vi "FN.vi"(0 "Offset_h":dbl, 1 "Offset_out":dbl, 2 "Inputs":dbl[](array[numeric]), 3 "Weights_h":dbl[][](array[numeric]), 4 "Weights_out":dbl[][](array[numeric])) -> (5 "Outputs_hx":dbl[](array[numeric]), 6 "Outputs_out":dbl[](array[numeric]))   [LabVIEW 2016]
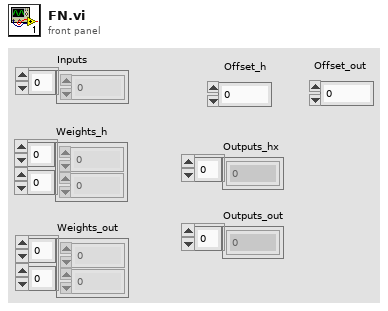
[diagram p1: front panel]
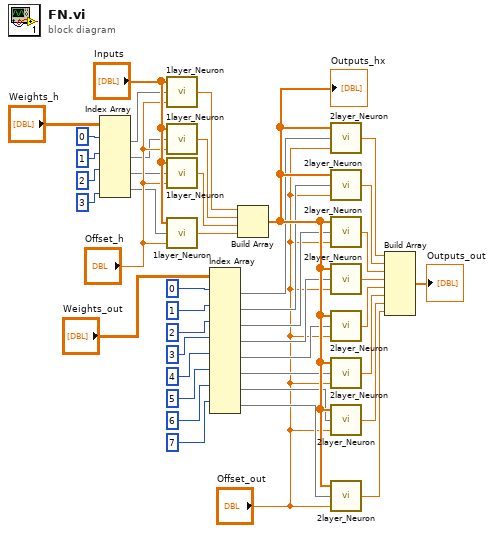
[diagram p0: block diagram]
diagram:
  n1 = Index Array(array="Weights_h", index (row) #1=0 ("index (row)"), index (row) #2=1 ("index (row)"), index (row) #3=2 ("index (row)"), index (col) #4=3 ("disabled index (col)")) -> (element #1=w31:dbl[], element #2=w30:dbl[], element #3=w29:dbl[], element #4=w28:dbl[])  [unwired: 4 in]
  n2 = call "1layer_Neuron.vi"("Offset"="Offset_h", "Weights"=w31, "Inputs"="Inputs") -> ("Output"=w41:dbl)
  n3 = call "1layer_Neuron.vi"("Offset"="Offset_h", "Weights"=w30, "Inputs"="Inputs") -> ("Output"=w40:dbl)
  n4 = call "1layer_Neuron.vi"("Offset"="Offset_h", "Weights"=w29, "Inputs"="Inputs") -> ("Output"=w39:dbl)
  n5 = call "1layer_Neuron.vi"("Offset"="Offset_h", "Weights"=w28, "Inputs"="Inputs") -> ("Output"=w38:dbl)
  n6 = Index Array(array="Weights_out", index (row) #1=0 ("index (row)"), index (row) #2=1 ("index (row)"), index (row) #3=2 ("index (row)"), index (row) #4=3 ("disabled index (col)"), index (row) #5=4 ("index (row)"), index (row) #6=5 ("index (row)"), index (row) #7=6 ("index (row)"), index (row) #8=7 ("disabled index (col)")) -> (element #1=w18:dbl[], element #2=w17:dbl[], element #3=w16:dbl[], element #4=w15:dbl[], element #5=w14:dbl[], element #6=w13:dbl[], element #7=w12:dbl[], element #8=w11:dbl[])  [unwired: 8 in]
  n7 = Build Array(w41, w40, w39, w38) -> (w37:dbl[])
  "Outputs_hx" <- w37
  n8 = call "2layer_Neuron.vi"("Offset"="Offset_out", "Weights_2layer"=w18, "Array_Out_hx"=w37) -> ("Output"=w8:dbl)
  n9 = call "2layer_Neuron.vi"("Offset"="Offset_out", "Weights_2layer"=w17, "Array_Out_hx"=w37) -> ("Output"=w7:dbl)
  n10 = call "2layer_Neuron.vi"("Offset"="Offset_out", "Weights_2layer"=w16, "Array_Out_hx"=w37) -> ("Output"=w6:dbl)
  n11 = call "2layer_Neuron.vi"("Offset"="Offset_out", "Weights_2layer"=w15, "Array_Out_hx"=w37) -> ("Output"=w5:dbl)
  n12 = call "2layer_Neuron.vi"("Offset"="Offset_out", "Weights_2layer"=w14, "Array_Out_hx"=w37) -> ("Output"=w4:dbl)
  n13 = call "2layer_Neuron.vi"("Offset"="Offset_out", "Weights_2layer"=w13, "Array_Out_hx"=w37) -> ("Output"=w3:dbl)
  n14 = call "2layer_Neuron.vi"("Offset"="Offset_out", "Weights_2layer"=w12, "Array_Out_hx"=w37) -> ("Output"=w2:dbl)
  n15 = call "2layer_Neuron.vi"("Offset"="Offset_out", "Weights_2layer"=w11, "Array_Out_hx"=w37) -> ("Output"=w1:dbl)
  n16 = Build Array(w8, w7, w6, w5, w4, w3, w2, w1) -> (→"Outputs_out":dbl[])
